vi "FVI_TRajectoire_rotation avec boussole.vi"() -> ()   [LabVIEW 2018]
uses:
  SwerveDrive.ctl
  <vilib>/Analysis/coordinate.llb/Angle Range (Degree).ctl
  <vilib>/Analysis/coordinate.llb/Angle Units.ctl
  <vilib>/Analysis/coordinate.llb/Wrap Angle (scalar).vi
  <vilib>/Analysis/coordinate.llb/Angle Rotation (scalar).vi
  MyGlobal.vi
  <vilib>/addons/control/pid/pid.llb/PID (DBL).vi
  <vilib>/addons/control/pid/NI_PID_pid.lvlib
  <vilib>/Analysis/NI_AAL_Angle.lvlib
panel:
  in  "Rotation":dbl format="%#_13g"
  in  "TSwerveDrive":T1
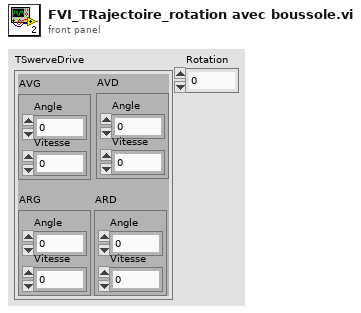
[diagram p1: front panel]
types:
  T1 = typedef "SwerveDrive.ctl" = cluster{"AVD":cluster{"Angle":dbl, "Vitesse":dbl}, "AVG":cluster{"Angle":dbl, "Vitesse":dbl}, "ARG":cluster{"Angle":dbl, "Vitesse":dbl}, "ARD":cluster{"Angle":dbl, "Vitesse":dbl}}
  T2 = typedef "NI_AAL_Angle.lvlib/Angle Units.ctl" = i32
  T3 = typedef "NI_AAL_Angle.lvlib/Angle Range (Degree).ctl" = u16
  T4 = cluster{"proportional gain (Kc)":dbl, "integral time (Ti, min)":dbl, "derivative time (Td, min)":dbl}
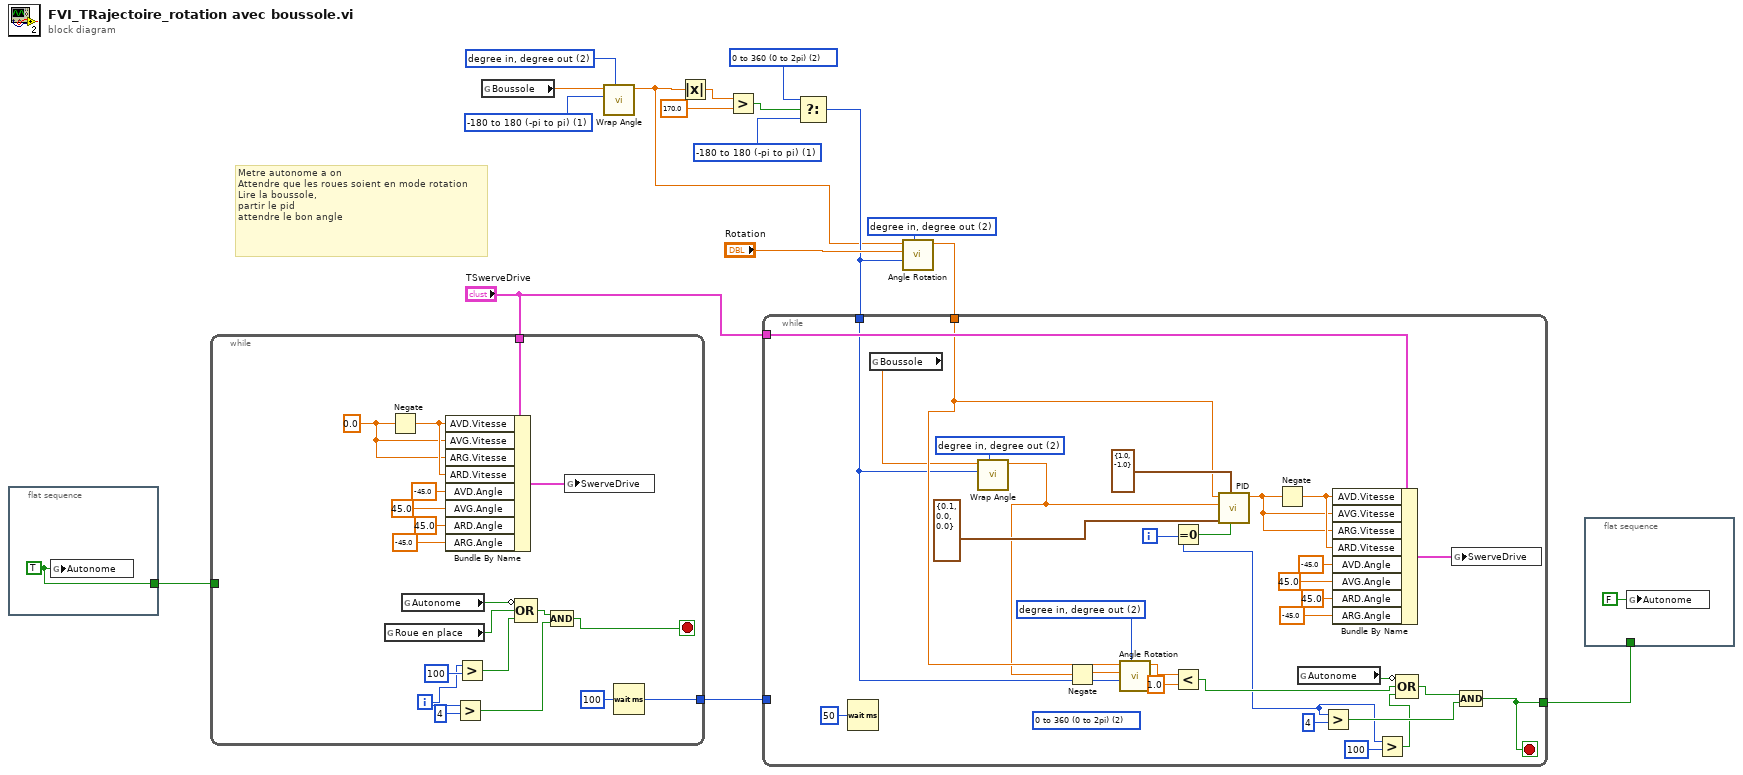
[diagram p0: block diagram]
diagram:
  w4 = T2 2 items=["radian in, radian out", "radian in, degree out", "degree in, degree out", "degree in, radian out"] ("angle units")
  w5 = T3 1 items=["none", "-180 to 180 (-pi to pi)", "0 to 360 (0 to 2pi)"] ("angle range")
  w6 = T3 2 items=["none", "-180 to 180 (-pi to pi)", "0 to 360 (0 to 2pi)"] ("angle range")
  w10 = T3 1 items=["none", "-180 to 180 (-pi to pi)", "0 to 360 (0 to 2pi)"] ("angle range")
  w16 = T2 2 items=["radian in, radian out", "radian in, degree out", "degree in, degree out", "degree in, radian out"] ("angle units")
  # "Metre autonome a on\nAttendre que les roues soient en mode rotation\nLire la boussole,\npartir le pid\nattendre le bon angle"
  n1 = flat-sequence {
    tunnel: [w18] -> w17
    frame #0 {
      w18 = TRUE ("Autonome")
      n2 = global write "MyGlobal.vi" "Autonome"(w18) -> ()
    }
  }
  n3 = while {
    tunnel: "TSwerveDrive" -> [w32]
    tunnel: w17 -> [_]
    tunnel: [w19] -> w12
    i -> [w23]
    stop <- w21 stop-if-true
    w31 = 0.0 ("x")
    n4 = global read "MyGlobal.vi" "Roue en place"() -> (w28:bool)
    n5 = Negate(x=w31) -> (-x=w33:dbl)
    n6 = global read "MyGlobal.vi" "Autonome"() -> (w29:bool)
    n7 = Bundle By Name(cluster=w32, "AVD.Vitesse"=w33, "AVG.Vitesse"=w31, "ARG.Vitesse"=w31, "ARD.Vitesse"=w33, "AVD.Angle"=-45.0, "AVG.Angle"=45.0, "ARD.Angle"=45.0, "ARG.Angle"=-45.0) -> (w30:T1)
    n8 = Greater?(x=w23, y=4) -> (0:w25:bool)
    n9 = Greater?(x=w23, y=100) -> (0:w22:bool)
    n10 = Compound Arithmetic op=OR(invert w29, w28, w22) -> (w26:bool)
    n11 = Compound Arithmetic op=AND(w26, w25) -> (w21:bool)
    n12 = global write "MyGlobal.vi" "SwerveDrive"(w30) -> ()
    n13 = Wait (ms)(milliseconds to wait=u32 100) -> (millisecond timer value=w19:u32)
  }
  n14 = global read "MyGlobal.vi" "Boussole"() -> (w11:dbl)
  n15 = call-poly <vilib>:"Wrap Angle.vi"("angle units"=w4, "angle range"=w10, "angle in"=w11) -> ("angle out"=w2:dbl)  [unwired: 7 in, 1 out]
  n16 = Absolute Value(x=w2) -> (abs(x)=w9:dbl)
  n17 = Greater?(x=w9, y=170.0) -> (0:w7:bool)
  n18 = Select(t=w6, s=w7, f=w5) -> (s? t:f=w3:T3)
  n19 = call-poly <vilib>:"Angle Rotation.vi"("angle units"=w16, "rotated angle range"=w3, "counterclockwise rotation"="Rotation", "angle"=w2) -> ("rotated angle"=w15:dbl)  [unwired: 6 in, 1 out]
  n20 = while {
    tunnel: w15 -> [w54]
    tunnel: "TSwerveDrive" -> [w58]
    tunnel: w12 -> [_]
    tunnel: w3 -> [w40]
    tunnel: [w38] -> w1
    i -> [w44]
    stop <- w38 stop-if-true
    w42 = T2 2 items=["radian in, radian out", "radian in, degree out", "degree in, degree out", "degree in, radian out"] ("angle units")
    (unwired) T3 2 items=["none", "-180 to 180 (-pi to pi)", "0 to 360 (0 to 2pi)"] ("rotated angle range")
    w55 = T2 2 items=["radian in, radian out", "radian in, degree out", "degree in, degree out", "degree in, radian out"] ("angle units")
    n21 = Wait (ms)(milliseconds to wait=u32 50) -> ()  [unwired: 1 out]
    n22 = global read "MyGlobal.vi" "Boussole"() -> (w41:dbl)
    n23 = call-poly <vilib>:"Wrap Angle.vi"("angle units"=w42, "angle range"=w40, "angle in"=w41) -> ("angle out"=w39:dbl)  [unwired: 7 in, 1 out]
    n24 = Negate(x=w39) -> (-x=w51:dbl)
    n25 = call-poly <vilib>:"Angle Rotation.vi"("angle units"=w55, "rotated angle range"=w40, "counterclockwise rotation"=w51, "angle"=w54) -> ("rotated angle"=w53:dbl)  [unwired: 6 in, 1 out]
    n26 = Equal To 0?(x=w44) -> (x = 0?=w66:bool)
    n27 = Less?(x=w53, y=1.0) -> (x < y?=w46:bool)
    n28 = call-poly <vilib>:"PID.vi"("reinitialize? (F)"=w66, "output range"=cluster{"output high":dbl, "output low":dbl} {"output high"=1.0, "output low"=-1.0}, "PID gains"=T4 {"proportional gain (Kc)"=0.1, "integral time (Ti, min)"=0.0, "derivative time (Td, min)"=0.0}, "process variable"=w39, "setpoint"=w54) -> ("output"=w57:dbl)  [unwired: 5 in, 1 out]
    n29 = Negate(x=w57) -> (-x=w63:dbl)
    n30 = global read "MyGlobal.vi" "Autonome"() -> (w50:bool)
    n31 = Greater?(x=w44, y=4) -> (0:w48:bool)
    n32 = Bundle By Name(cluster=w58, "AVD.Vitesse"=w63, "AVG.Vitesse"=w57, "ARG.Vitesse"=w57, "ARD.Vitesse"=w63, "AVD.Angle"=-45.0, "AVG.Angle"=45.0, "ARD.Angle"=45.0, "ARG.Angle"=-45.0) -> (w64:T1)
    n33 = Greater?(x=w44, y=100) -> (0:w43:bool)
    n34 = Compound Arithmetic op=OR(invert w50, w46, w43) -> (w47:bool)
    n35 = global write "MyGlobal.vi" "SwerveDrive"(w64) -> ()
    n36 = Compound Arithmetic op=AND(w47, w48) -> (w38:bool)
  }
  n37 = flat-sequence {
    tunnel: w1 -> [_]
    frame #0 {
      n38 = global write "MyGlobal.vi" "Autonome"(FALSE ("Autonome")) -> ()
    }
  }
